vi "add_object.vi"(6 "wait for reply (T)":bool=TRUE, 7 "position_y":i32, 8 "error in":errorcluster, 9 "object_name":string, 10 "diagram_id":i32, 11 "position_x":i32) -> (0 "error out":errorcluster, 1 "timed out?":bool, 2 "result":string, 3 "object_id":i32)   [LabVIEW 2025, in "Scripting Server.lvlib"]
doc: "Adds an object to the block diagram, structure sub-diagram or frontpanel of the referenced vi. Get a VI reference from new_vi or get a structure sub-diagram by get_stucture_diagram to add to this. If adding a control, consider the create_control tool and think about adding objects first and then creating structures around them using the enclose with selection."
uses:
  Scripting Server.lvlib
  Add Object Argument--cluster.ctl
  Add Object (Reply Payload)--cluster.ctl
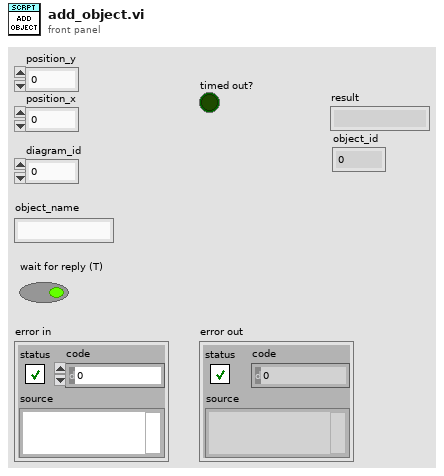
[diagram p1: front panel]
types:
  T1 = typedef "Scripting Server.lvlib/Add Object Argument--cluster.ctl" = cluster{"VI Reference":i32, "Object Name":string, "Wait Notifier":refnum<notifier>, "wait for reply":bool, "position_x":i32, "position_y":i32}
  T2 = typedef "Scripting Server.lvlib/Request Events--cluster.ctl" = cluster{"Stop Module":refnum<user-event>, "Show Panel":refnum<user-event>, "Hide Panel":refnum<user-event>, "Get Module Execution Status":refnum<user-event>, "Show Diagram":refnum<user-event>, "New VI":refnum<user-event>, "Add Object":refnum<user-event>, "Connect Objects":refnum<user-event>, "Get Object Terminals":refnum<user-event>, "get vi error list":refnum<user-event>, "Cleanup VI":refnum<user-event>, "create_control":refnum<user-event>, "Run VI":refnum<user-event>, "add_to_selection":refnum<user-event>, "clear_selection_list":refnum<user-event>, "remove_from_selection":refnum<user-event>, "enclose_selection":refnum<user-event>, "rename_object":refnum<user-event>, "set_value":refnum<user-event>, "delete_object":refnum<user-event>, "save_vi":refnum<user-event>, "get_structure_diagram":refnum<user-event>, "add_subvi":refnum<user-event>, "connect_to_pane":refnum<user-event>, "get_object_help":refnum<user-event>, "get_loop_conditional_terminal":refnum<user-event>, "show_conditional_terminal":refnum<user-event>, "get_loop_iteration_terminal":refnum<user-event>, "Read Config Data":refnum<user-event>, "get_allowed_paths":refnum<user-event>, "create_project":refnum<user-event>, "Set Allowed Paths":refnum<user-event>, "open_vi":refnum<user-event>, "Private.Register MCP Events":refnum<user-event>, "New MCP RPC Message":refnum<user-event>, "get-available-objects":refnum<user-event>}
  T3 = typedef "Scripting Server.lvlib/Add Object (Reply Payload)--cluster.ctl" = cluster{"error":errorcluster, "Object ID":i32, "Result":string}
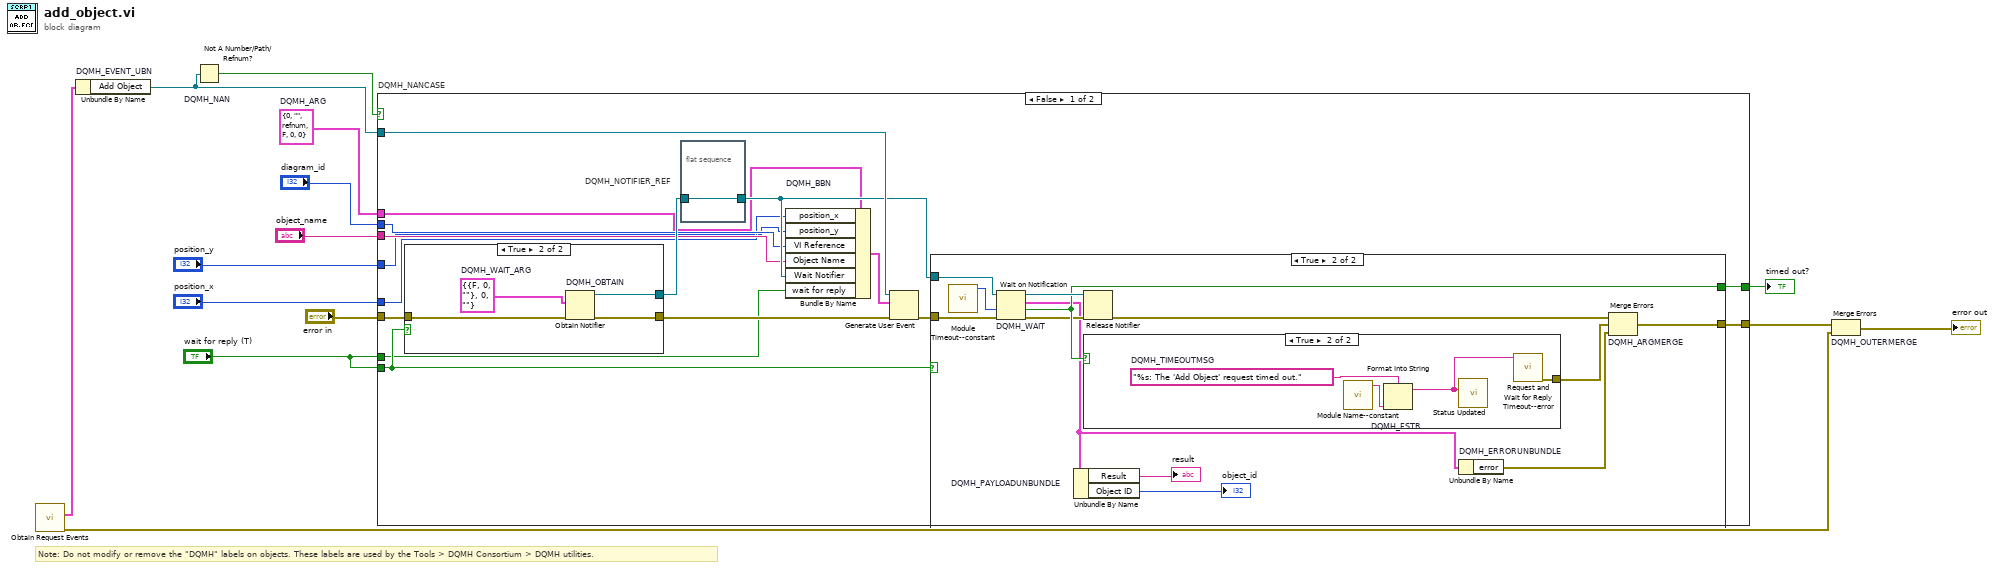
[diagram p0: block diagram]
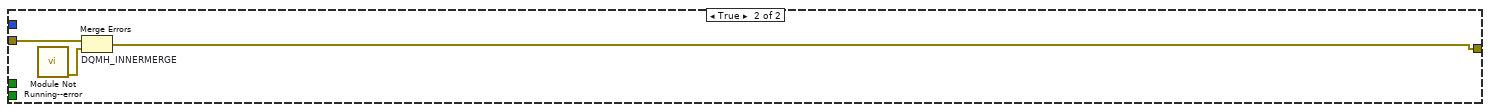
[diagram p5: hidden frame]
diagram:
  w8 = T1 {"VI Reference"=0, "Object Name"="", "Wait Notifier"=refnum, "wait for reply"=FALSE, "position_x"=0, "position_y"=0}  # DQMH_ARG
  # "Note: Do not modify or remove the \"DQMH\" labels on objects. These labels are used by the Tools > DQMH Consortium > DQMH utilities."
  n1 = call "Obtain Request Events.vi"() -> ("error out"=w4:errorcluster, "Scripting Server Request Events"=w3:T2)  [unwired: 10 in]
  n2 = Unbundle By Name "DQMH_EVENT_UBN"(w3) -> ("Add Object"=w9:refnum<user-event>)
  n3 = Not A Number/Path/Refnum? "DQMH_NAN"(number/path/refnum=w9) -> (NaN/Path/Refnum?=w10:bool)
  n4 = case "DQMH_NANCASE" shown="False" w10 {
    tunnel: "error in" -> [w30 w57]
    tunnel: w9 -> [w28 _]
    tunnel: [w25 w56] -> w11
    tunnel: [w26 _] -> w13
    tunnel: "wait for reply (T)" -> [w23 _]
    tunnel: w8 -> [w20 _]
    tunnel: "diagram_id" -> [w19 _]
    tunnel: "object_name" -> [w18 _]
    tunnel: "wait for reply (T)" -> [w17 _]
    tunnel: "position_x" -> [w16 _]
    tunnel: "position_y" -> [w15 _]
    frame False {
      n5 = case shown="True" w23 {
        tunnel: w30 -> [w50 w54]
        tunnel: [w50 w53] -> w27
        tunnel: [_ w51] -> w22
        frame False {
        }
        frame True {
          w52 = T3 {"error"={"status"=FALSE, "code"=0, "source"=""}, "Object ID"=0, "Result"=""}  # DQMH_WAIT_ARG
          n6 = Obtain Notifier "DQMH_OBTAIN"(notification data type=w52, error in (no error)=w54) -> (notifier out=w51:refnum<notifier>, error out=w53:errorcluster)  [unwired: 2 in, 1 out]
        }
      }
      n7 = flat-sequence "DQMH_NOTIFIER_REF" {
        tunnel: w22 -> [w31]
        tunnel: [w31] -> w21
        frame #0 {
        }
      }
      n8 = Bundle By Name "DQMH_BBN"(cluster=w20, "position_x"=w16, "position_y"=w15, "VI Reference"=w19, "Object Name"=w18, "Wait Notifier"=w21, "wait for reply"=w17) -> (w24:T1)
      n9 = Generate User Event(user event=w28, event data cluster=w24, error in=w27) -> (error out=w29:errorcluster)  [unwired: 1 in, 1 out]
      n10 = case shown="True" w23 {
        tunnel: w29 -> [w32 w45]
        tunnel: w21 -> [_ w44]
        tunnel: [_ w42] -> w26
        tunnel: [w32 w41] -> w25
        frame False {
        }
        frame True {
          n11 = call "Module Timeout--constant.vi"() -> ("Module Timeout"=w35:i32)  [unwired: 11 in]
          n12 = Wait on Notification "DQMH_WAIT"(notifier=w44, timeout in ms (-1)=w35, error in (no error)=w45) -> (notifier out=w43:refnum<notifier>, notification=w36:T3, timed out?=w42:bool, error out=w40:errorcluster)  [unwired: 1 in]
          n13 = Unbundle By Name "DQMH_PAYLOADUNBUNDLE"(w36) -> ("Result"=→"result":string, "Object ID"=→"object_id":i32)
          n14 = Release Notifier(notifier=w43, error in (no error)=w40) -> (error out=w39:errorcluster)  [unwired: 1 in, 2 out]
          n15 = case shown="True" w42 {
            tunnel: [_ w47] -> w37
            frame False {
            }
            frame True {
              w49 = "%s: The 'Add Object' request timed out."  # DQMH_TIMEOUTMSG
              n16 = call "Module Name--constant.vi"() -> ("Module Name"=w46:string)  [unwired: 11 in]
              n17 = Format Into String "DQMH_FSTR"(format string=w49, w46) -> (resulting string=w48:string)  [unwired: 2 in, 1 out]
              n18 = call "Status Updated.vi"("Status"=w48) -> ()  [unwired: 10 in, 1 out]
              n19 = call "Request and Wait for Reply Timeout--error.vi"("Error Message"=w48) -> ("error out"=w47:errorcluster)  [unwired: 10 in]
            }
          }
          n20 = Unbundle By Name "DQMH_ERRORUNBUNDLE"(w36) -> ("error"=w38:errorcluster)
          n21 = Merge Errors "DQMH_ARGMERGE"(w39, w37, w38) -> (w41:errorcluster)
        }
      }
    }
    frame True {
      n22 = call "Module Not Running--error.vi"() -> ("error out"=w55:errorcluster)  [unwired: 11 in]
      n23 = Merge Errors "DQMH_INNERMERGE"(w57, w55) -> (w56:errorcluster)
    }
  }
  "timed out?" <- w13
  n24 = Merge Errors "DQMH_OUTERMERGE"(w11, w4) -> (→"error out":errorcluster)
